vi "Read Read Delay.vi"(8 "error in (no error)":errorcluster, 11 "Dashboard Server in":refnum<class "Dashboard Server.lvclass">) -> (0 "error out":errorcluster, 2 "Read Delay":u32, 3 "Dashboard Server out":refnum<class "Dashboard Server.lvclass">)   [LabVIEW 2016, in "Dashboard Server.lvclass"]
uses:
  Dashboard Server.lvclass
  Dashboard Server.lvclass/Dashboard Server.ctl
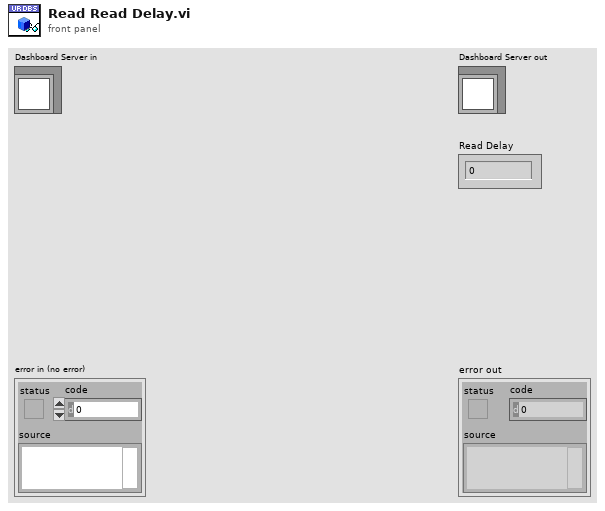
[diagram p1: front panel]
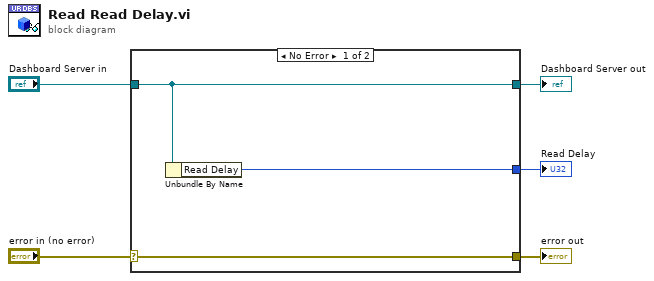
[diagram p0: block diagram]
diagram:
  n1 = case shown="No Error" "error in (no error)" {
    selector: "error in (no error)" -> [w8 w9]
    tunnel: [w8 w9] -> w4
    tunnel: [w7 w10] -> w2
    tunnel: "Dashboard Server in" -> [w7 w10]
    tunnel: [w6 _] -> w1
    frame No Error {
      n2 = Unbundle By Name(w7) -> ("Read Delay"=w6:u32)
    }
    frame Error {
    }
  }
  "error out" <- w4
  "Dashboard Server out" <- w2
  "Read Delay" <- w1
